vi "GetTerminalReference.vi"(8 "error in":errorcluster, 11 "Terminal in":refnum<class "Terminal.lvclass">) -> (0 "error out":errorcluster, 1 "reference":refnum<vi>, 3 "Terminal out":refnum<class "Terminal.lvclass">)   [LabVIEW 2014, in "Raspberry Pi Compatible Compiler for LabVIEW.lvlib" / "Terminal.lvclass"]
uses:
  Terminal.lvclass
  Generic/Generic.lvclass
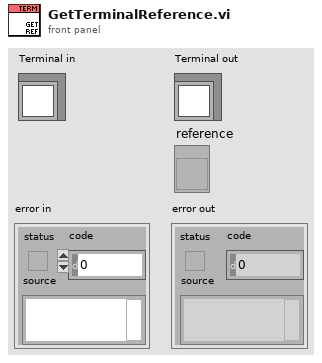
[diagram p1: front panel]
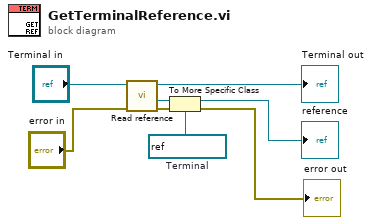
[diagram p0: block diagram]
diagram:
  w4 = refnum<vi> refnum  # Terminal
  n1 = call "Read reference.vi"("error in"="error in", "GObject in"="Terminal in") -> ("error out"=w5:errorcluster, "reference"=w6:refnum<vi>, "GObject out"=→"Terminal out":refnum<class "Terminal.lvclass">)  [unwired: 5 in]
  n2 = To More Specific Class(target class=w4, reference=w6, error in=w5) -> (specific class reference=→"reference":refnum<vi>, error out=→"error out":errorcluster)
